vi "run.vi"(8 "error in (no error)":errorcluster, 11 "StimulatorDL090824Gate in":refnum<class "StimulatorDL090824Gate.lvclass">) -> (0 "error out":errorcluster, 3 "StimulatorDL090824Gate out":refnum<class "StimulatorDL090824Gate.lvclass">)   [LabVIEW 2010, in "StimulatorDL090824Gate.lvclass"]
uses:
  StimulatorDL090824Gate.lvclass
  GenericStimulator/GenericStimulator/GenericStimulator.lvclass
  common/classes/ErrorController/ErrorController/ErrorController.lvclass
  StimulatorDL090724Scaffold/StimulatorDL090724Scaffold/Stimulator090724Scaffold.lvclass
  Clock/GenericClock/GenericClock/GenericClock.lvclass
  main/labview_source/controls/undock_button.ctl
panel:
  in  "button:undock":T1
  in  "Tab Control":enum32{"User", "Debug", "About"}(tab)
  in  "repetitions":i32=1
  in  "repetition period":dbl[unit]
  in  "offset":dbl[unit]
  in  "pulse duration":dbl[unit]=1.0
  out "finished?":bool
  # "StimulatorDL090824Gate"
  # "Implemented by: \nDominik Langer, University of Zurich"
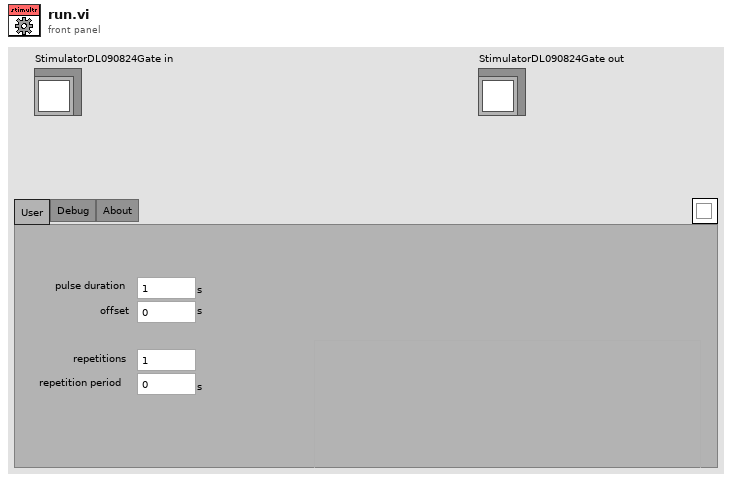
[diagram p1: front panel]
types:
  T1 = typedef "undock_button.ctl" = bool
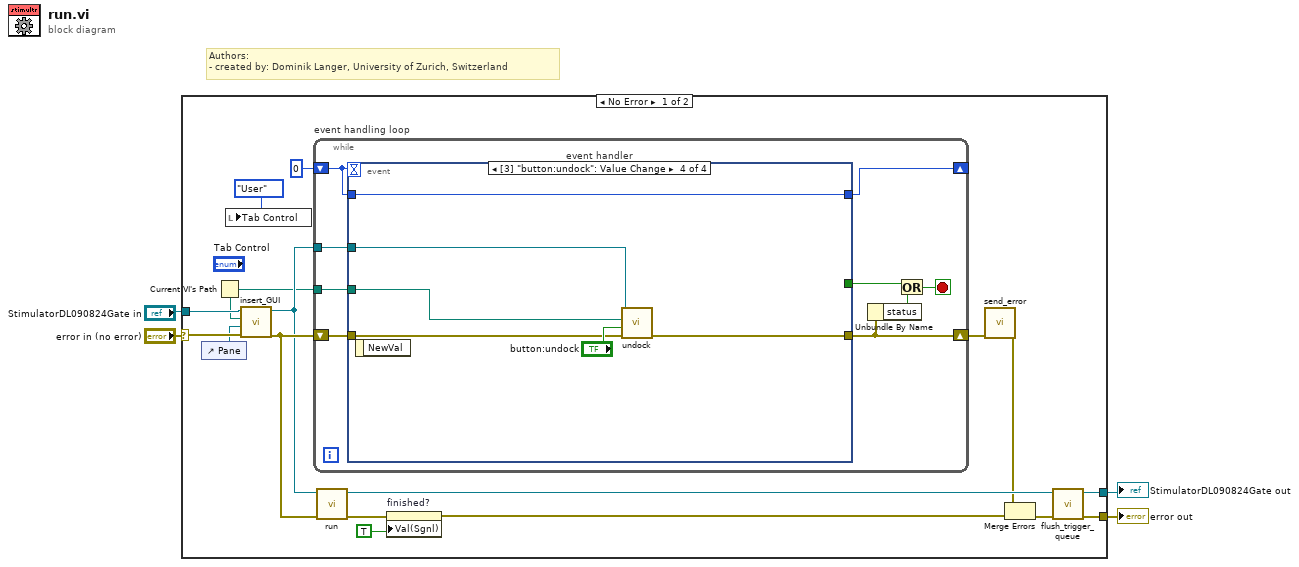
[diagram p0: block diagram]
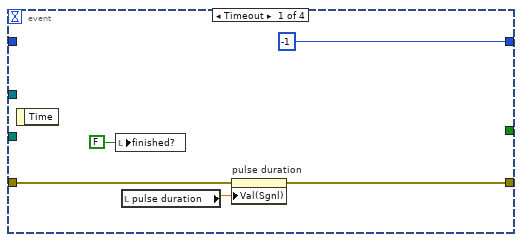
[diagram p2: hidden frame]
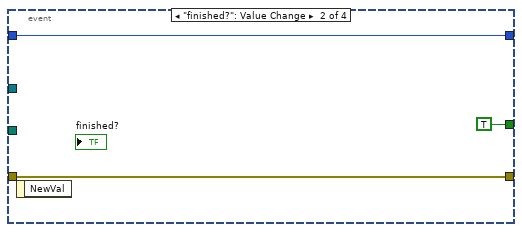
[diagram p3: hidden frame]
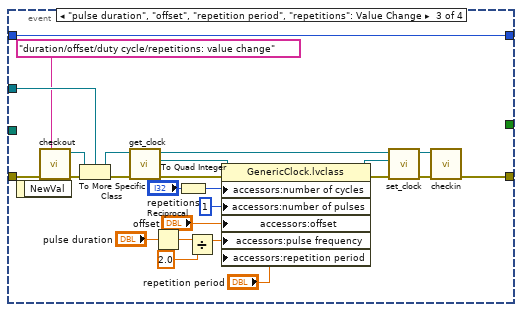
[diagram p4: hidden frame]
diagram:
  # "Authors: \n- created by: Dominik Langer, University of Zurich, Switzerland"
  n1 = case shown="No Error" "error in (no error)" {
    selector: "error in (no error)" -> [w16 w70]
    tunnel: "StimulatorDL090824Gate in" -> [w15 w71]
    tunnel: [w8 w71] -> w1
    tunnel: [w9 w70] -> w2
    frame No Error {
      n2 = control-ref of="Pane"() -> (w12:refnum<vi>)
      n3 = Current VI's Path() -> (path=w5:path)
      n4 = local write "Tab Control"(enum32{"User", "Debug", "About"}."User" ("Tab Control")) -> ()
      n5 = call-dynamic "insert_GUI.vi"("error in (no error)"=w16, "Pane"=w12, "VI path"=w5, "GenericComponent in"=w15) -> ("error out"=w17:errorcluster, "GenericComponent out"=w14:refnum<class "StimulatorDL090824Gate.lvclass">)  [unwired: 6 in]
      n6 = while "event handling loop" {
        shift-right: [w26] -> w7
        shift-left: w17 -> [w30]
        tunnel: w14 -> [w29]
        shift-right: [w27] -> _
        shift-left: 0 -> [w28]
        tunnel: w5 -> [w22]
        stop <- w23 stop-if-true
        n7 = event "event handler" shown="[3] \"button:undock\": Value Change" {
          selector: _ -> [_ _ _ _]
          dyn-events: _ -> [_ _ _ _]
          timeout: w28 -> [_ _ _ _]
          tunnel: w30 -> [w33 w37 w62 w67]
          tunnel: w29 -> [_ _ w60 w65]
          tunnel: [-1 w38 w63 w69] -> w27
          tunnel: w28 -> [_ w38 w63 w69]
          tunnel: [w32 w37 w44 w66] -> w26
          tunnel: [_ TRUE _ _] -> w24
          tunnel: w22 -> [_ _ _ w64]
          event Timeout {
            n8 = event-data() -> ()  [unwired: 1 in, 1 out]
            n9 = local write "finished?"(FALSE ("finished?")) -> ()
            n10 = local read "pulse duration"() -> (w31:dbl[unit])
            n11 = property on="pulse duration" class="DigNum (strict)"(error in=w33, "Val(Sgnl)"=w31) -> (error out=w32:errorcluster)  [unwired: 1 in, 1 out]
          }
          event "finished?": Value Change {
            n12 = event-data() -> ()  [unwired: 1 in, 1 out]
          }
          event "pulse duration", "offset", "repetition period", "repetitions": Value Change {
            n13 = event-data() -> ()  [unwired: 1 in, 1 out]
            n14 = call "checkout.vi"("locked by?"="duration/offset/duty cycle/repetitions: value change", "error in (no error)"=w62) -> ("error out"=w61:errorcluster, "GenericStimulator out"=w59:refnum<class "GenericStimulator.lvclass">)  [unwired: 8 out]
            n15 = To More Specific Class(target class=w60, reference=w59, error in=w61) -> (specific class reference=w56:refnum<class "StimulatorDL090824Gate.lvclass">, error out=w57:errorcluster)
            n16 = call "get_clock.vi"("error in (no error)"=w57, "Stimulator090724Scaffold in"=w56) -> ("error out"=w54:errorcluster, "clock"=w55:refnum<class "GenericClock.lvclass">, "Stimulator090724Scaffold out"=w48:refnum<class "StimulatorDL090824Gate.lvclass">)  [unwired: 7 in]
            n17 = Reciprocal(x="pulse duration") -> (1/x=w41:dbl[unit])
            n18 = To Quad Integer(1:"repetitions") -> (0:w50:i64)
            n19 = Divide(x=w41, y=2.0) -> (x/y=w39:dbl[unit])
            n20 = property class="GenericClock.lvclass"(reference=w55, error in=w54, "accessors:number of cycles"=w50, "accessors:number of pulses"=i64 1 ("number of pulses"), "accessors:offset"="offset", "accessors:pulse frequency"=w39, "accessors:repetition period"="repetition period") -> (reference out=w47:refnum<class "GenericClock.lvclass">, error out=w49:errorcluster)
            n21 = call-dynamic "set_clock.vi"("error in (no error)"=w49, "clock"=w47, "Stimulator090724Scaffold in"=w48) -> ("error out"=w45:errorcluster, "Stimulator090724Scaffold out"=w46:refnum<class "StimulatorDL090824Gate.lvclass">)  [unwired: 7 in]
            n22 = call-dynamic "checkin.vi"("error in (no error)"=w45, "GenericStimulator in"=w46) -> ("error out"=w44:errorcluster)  [unwired: 8 in, 1 out]
          }
          event Value Change {
            n23 = event-data() -> ()  [unwired: 1 in, 1 out]
            n24 = call-dynamic "undock.vi"("error in (no error)"=w67, "undock?"="button:undock", "VI path"=w64, "component in"=w65) -> ("error out"=w66:errorcluster)  [unwired: 6 in, 1 out]
          }
        }
        n25 = Unbundle By Name(w26) -> ("status"=w25:bool)
        n26 = Or(x=w24, y=w25) -> (x .or. y?=w23:bool)
      }
      n27 = call-parent "run.vi"("error in (no error)"=w17, "Stimulator090724Scaffold in"=w14) -> ("error out"=w19:errorcluster, "Stimulator090724Scaffold out"=w11:refnum<class "StimulatorDL090824Gate.lvclass">)  [unwired: 8 in]
      n28 = property on="finished?" class="Bool (strict)"(error in=w19, "Val(Sgnl)"=TRUE ("Value (Signaling)")) -> (error out=w18:errorcluster)  [unwired: 1 in, 1 out]
      n29 = call "send_error.vi"("error in (no error)"=w7) -> ("error out"=w6:errorcluster)  [unwired: 10 in]
      n30 = Merge Errors(w6, w18) -> (w10:errorcluster)
      n31 = call-dynamic "flush_trigger_queue.vi"("error in (no error)"=w10, "GenericToplevelComponent in"=w11) -> ("error out"=w9:errorcluster, "GenericToplevelComponent out"=w8:refnum<class "StimulatorDL090824Gate.lvclass">)  [unwired: 8 in]
    }
    frame Error {
    }
  }
  "error out" <- w2
  "StimulatorDL090824Gate out" <- w1
